vi "Decode_Arduino_Trame.vi"(0 "arduinoData":string, 11 "adressable?":bool=TRUE) -> (4 "address":string, 6 "function":string, 10 "parameter":string, 14 "dataOut":T1)   [LabVIEW 2024]
uses:
  cluster_DataArduino.ctl
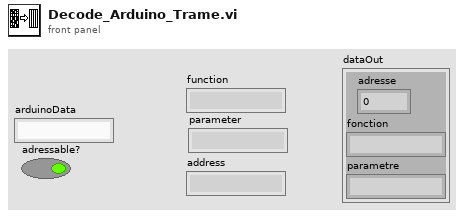
[diagram p1: front panel]
types:
  T1 = typedef "cluster_DataArduino.ctl" = cluster{"adresse":i32, "fonction":string, "parametre":string}
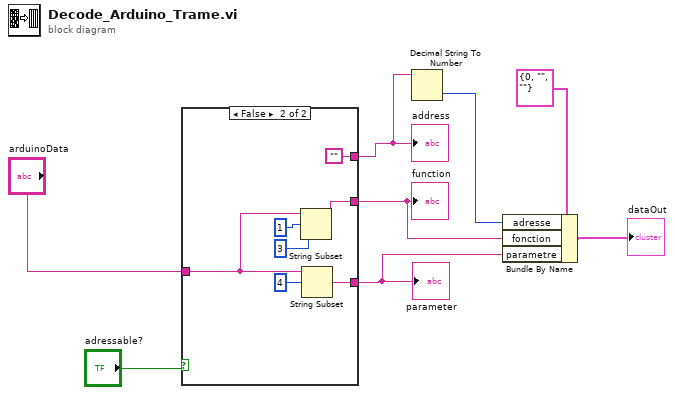
[diagram p0: block diagram]
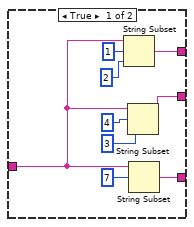
[diagram p2: hidden frame]
diagram:
  n1 = case shown="False" "adressable?" {
    tunnel: [w14 w21] -> w5
    tunnel: [w13 w20] -> w6
    tunnel: "arduinoData" -> [w12 w19]
    tunnel: [w9 "" ("arduinoData")] -> w4
    frame True {
      n2 = String Subset(string=w12, offset (0)=1, length (rest)=2 ("offset (0)")) -> (substring=w9:string)
      n3 = String Subset(string=w12, offset (0)=4, length (rest)=3 ("longueur (reste)")) -> (substring=w14:string)
      n4 = String Subset(string=w12, offset (0)=7) -> (substring=w13:string)  [unwired: 1 in]
    }
    frame False {
      n5 = String Subset(string=w19, offset (0)=1, length (rest)=3 ("longueur (reste)")) -> (substring=w21:string)
      n6 = String Subset(string=w19, offset (0)=4) -> (substring=w20:string)  [unwired: 1 in]
    }
  }
  "function" <- w5
  "parameter" <- w6
  "address" <- w4
  n7 = Decimal String To Number(string=w4) -> (number=w3:i32)  [unwired: 2 in, 1 out]
  n8 = Bundle By Name(cluster=T1 {"adresse"=0, "fonction"="", "parametre"=""} ("clusterDataArduino"), "adresse"=w3, "fonction"=w5, "parametre"=w6) -> (→"dataOut":T1)
